vi "debug_csv_graph_values.vi"(3 "error in":errorcluster, 4 "Value Distance/Load":string[](array[string]), 5 "Enum":enum16{"Int", "Update"}(ring)=enum."Update") -> (0 "error our":errorcluster, 2 "appended path 2":path)   [LabVIEW 2017]
doc: "VI for saving Hardware setting for PLC IP and Camera IP address. an PORT"
uses:
  <vilib>/Utility/file.llb/Write Delimited Spreadsheet (string).vi
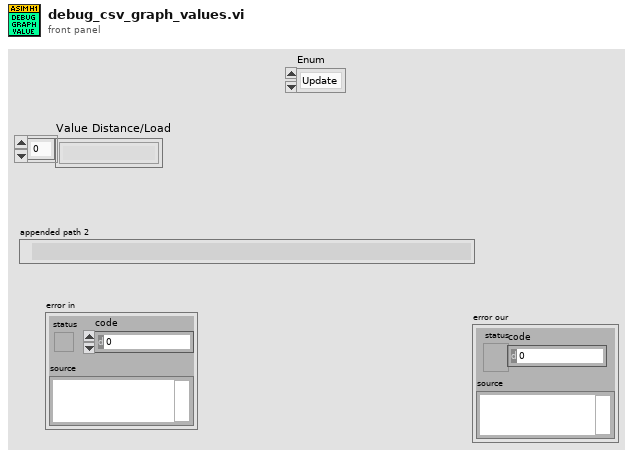
[diagram p1: front panel]
types:
  T1 = enum32{"invalid app kind", "Development System", "Run Time System", "Student Edition", "Embedded LabVIEW", "Evaluation", "Custom"}
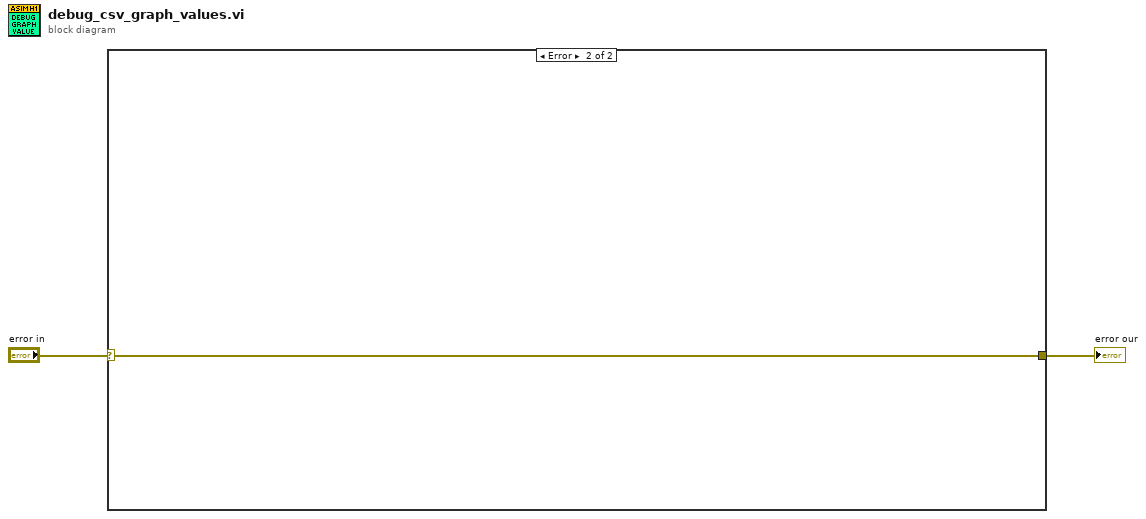
[diagram p0: block diagram]
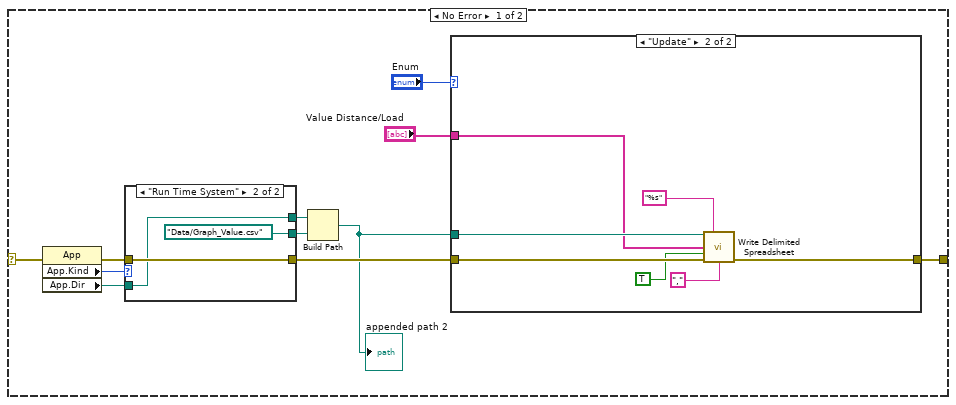
[diagram p2: hidden frame]
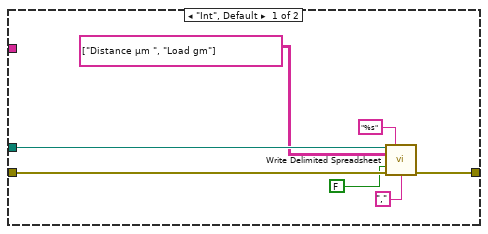
[diagram p3: hidden frame]
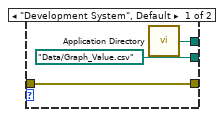
[diagram p4: hidden frame]
diagram:
  n1 = case shown="Error" "error in" {
    selector: "error in" -> [w6 w34]
    tunnel: [w12 w34] -> w2
    frame No Error {
      n2 = property class="App"(error in=w6) -> (error out=w10:errorcluster, "App.Kind"=w5:T1, "App.Dir"=w9:path)  [unwired: 1 in, 1 out]
      n3 = case shown="\"Run Time System\"" w5 {
        tunnel: [w30 w33] -> w11
        tunnel: w10 -> [w30 w33]
        tunnel: w9 -> [_ w31]
        tunnel: [path "Data/Graph_Value.csv" path "Data/Graph_Value.csv"] -> w8
        tunnel: [w28 w31] -> w7
        frame "Development System", Default {
          n4 = call <vilib>:"Application Directory.vi"() -> ("Application Directory"=w28:path)
        }
        frame "Run Time System" {
        }
      }
      n5 = Build Path(base path=w7, name or relative path=w8) -> (appended path=w4:path)
      "appended path 2" <- w4
      n6 = case shown="\"Update\"" "Enum" {
        tunnel: [w19 w25] -> w12
        tunnel: w11 -> [w20 w26]
        tunnel: w4 -> [w18 w27]
        tunnel: "Value Distance/Load" -> [_ w21]
        frame "Int", Default {
          n7 = call-poly <vilib>:"Write Delimited Spreadsheet.vi"("file path (dialog if empty)"=w18, "format (%s)"="%s", "2D data"=string[][] [["Distance µm ", "Load gm"]], "append to file? (new file:F)"=FALSE, "error in (no error)"=w20, "delimiter (\\t)"=",") -> ("error out"=w19:errorcluster)  [unwired: 8 in, 1 out]
        }
        frame "Update" {
          n8 = call-poly <vilib>:"Write Delimited Spreadsheet.vi"("file path (dialog if empty)"=w27, "format (%s)"="%s", "1D data"=w21, "append to file? (new file:F)"=TRUE, "error in (no error)"=w26, "delimiter (\\t)"=",") -> ("error out"=w25:errorcluster)  [unwired: 8 in, 1 out]
        }
      }
    }
    frame Error {
    }
  }
  "error our" <- w2
